vi "getcalpwr.vi"(5 "RF On":bool=TRUE, 7 "caldata":dbl[][](array[numeric]) format="%0.3f", 8 "RF HP":bool=TRUE, 9 "attn":dbl, 10 "freq":dbl=1000.0 min=34.375 max=4400.0 step=1.0 format="%_7g") -> (2 "actual":dbl)   [LabVIEW 2012]
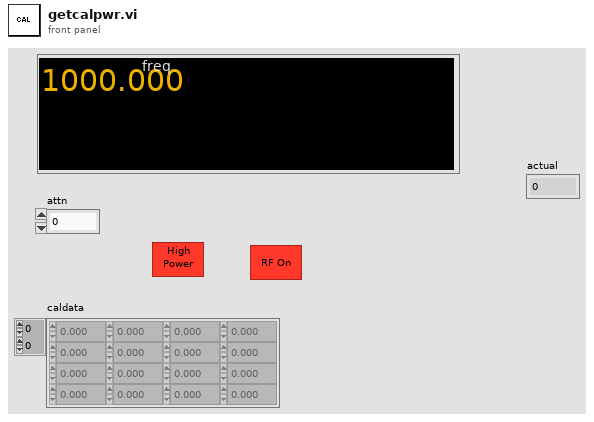
[diagram p1: front panel]
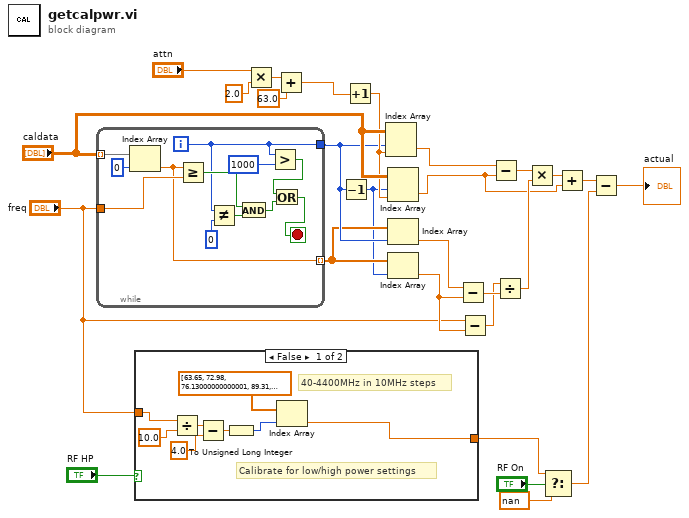
[diagram p0: block diagram]
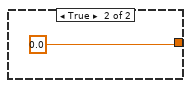
[diagram p2: hidden frame]
diagram:
  n1 = while {
    tunnel: "caldata" -> [w39] mode=indexing
    tunnel: "freq" -> [w37]
    tunnel: [w32] -> w25
    tunnel: [w33] -> w24 mode=indexing
    i -> [w32]
    stop <- w28 stop-if-true
    n2 = Index Array(array=w39, index=0) -> (element=w33:dbl)
    n3 = Greater Or Equal?(x=w33, y=w37) -> (x >= y?=w34:bool)
    n4 = Not Equal?(x=w32, y=0) -> (x != y?=w35:bool)
    n5 = And(x=w34, y=w35) -> (x .and. y?=w30:bool)
    n6 = Greater?(x=w32, y=1000) -> (0:w29:bool)
    n7 = Or(x=w29, y=w30) -> (x .or. y?=w28:bool)
  }
  n8 = case shown="False" "RF HP" {
    tunnel: [w40 0.0] -> w8
    tunnel: "freq" -> [w46 _]
    frame False {
      # "Calibrate for low/high power settings"
      # "40-4400MHz in 10MHz steps"
      n9 = Divide(x=w46, y=10.0) -> (x/y=w44:dbl)
      n10 = Subtract(x=w44, y=4.0) -> (x-y=w42:dbl)
      n11 = To Unsigned Long Integer(number=w42) -> (unsigned 32bit integer=w41:u32)
      n12 = Index Array(array=dbl[] [63.65, 72.98, 76.13000000000001, 89.31, 77.55000000000001, 78.89, 84.86, 81.81, 79.77000000000001, 80.12, 77.53, 78.39000000000001, 76.36, 76.32, 75.96, 74.75999999999999, 74.81, 74.34, 73.81, 73.35, 72.8, 72.87, 72.71000000000001, 71.77, 71.39, 71.28, 71.19, 70.59, 70.28, 69.9, 70.14999999999999, 69.73, 69.03, 69.1, 69.16, 68.39, 68.81, 67.9, 67.76, 67.55, 67.13, 67.02, 66.84, 66.67, 66.37, 66.11, 65.95, 65.74000000000001, 65.41, 65.23, 65.15, 64.83, 64.59, 64.46, 64.36, 64.14, 63.99, 63.79, 63.64, 63.53, 63.39, 63.18000000000001, 63.02, 62.88, 62.8, 62.63, 62.489999999999995, 62.349999999999994, 62.17999999999999, 62.019999999999996, 61.86, 61.699999999999996, 61.620000000000005, 61.53, 61.46, 61.3, 61.2, 61.120000000000005, 60.910000000000004, 60.730000000000004, 60.68, 60.56, 60.510000000000005, 60.440000000000005, 60.26, 59.98, 59.98, 59.8, 59.75, 59.589999999999996, 59.559999999999995, 59.43, 59.29, 59.290000000000006, 59.1, 59.019999999999996, 58.95, 58.92, 58.82, 58.82, 58.68, 58.52, 58.519999999999996, 58.56, 58.44, 58.32, 58.44, 58.349999999999994, 58.3, 58.25, 58.089999999999996, 58.0, 57.97, 57.97, 57.89, 57.86, 57.81999999999999, 57.769999999999996, 57.65, 57.510000000000005, 57.480000000000004, 57.38, 57.27, 57.26, 57.120000000000005, 57.089999999999996, 57.07, 57.07, 56.93, 56.85, 56.9, 56.84, 56.72, 56.74, 56.56, 56.44, 56.45, 56.35, 56.35, 56.3, 56.300000000000004, 56.330000000000005, 56.18, 55.989999999999995, 56.0, 55.83, 55.870000000000005, 56.0, 55.81, 55.53, 55.690000000000005, 55.85, 55.599999999999994, 55.36, 55.57, 55.86, 55.63, 55.24, 55.48, 55.72, 55.22, 55.56, 55.18000000000001, 54.790000000000006, 55.11, 54.79, 55.05, 54.72, 54.83, 54.93, 54.709999999999994, 54.48, 54.64, 54.53, 54.64, 54.53, 54.53, 54.42, 54.39, 54.339999999999996, 54.27, 54.34, 54.39, 54.25, 54.3, 54.22, 54.06, 54.089999999999996, 54.21, 54.31, 54.24, 54.14, 54.14, 54.11, 53.8, 53.830000000000005, 53.68, 53.53, 53.6, 53.519999999999996, 53.66, 53.47, 53.5, 53.410000000000004, 53.489999999999995, 53.510000000000005, 53.580000000000005, 53.550000000000004, 53.540000000000006, 53.49, 53.49, 53.34, 53.2, 53.17, 53.14, 53.080000000000005, 47.42, 47.03, 46.699999999999996, 46.56, 46.449999999999996, 46.31, 45.980000000000004, 45.89, 45.790000000000006, 45.739999999999995, 45.43, 45.120000000000005, 45.01, 44.89, 44.71, 44.33, 44.29, 44.120000000000005, 44.04, 43.72, 43.51, 43.480000000000004, 43.46, 43.39, 43.09, 42.96, 42.93, 42.93, 42.74, 42.44, 42.41, 42.48, 42.54, 42.4, 42.150000000000006, 42.17, 42.290000000000006, 42.31, 42.15, 41.96, 41.93, 41.89, 41.87, 41.71, 41.47, 41.48, 41.47, 41.45, 41.230000000000004, 40.89, 40.81, 40.67, 40.58, 40.5, 40.230000000000004, 40.04, 40.0, 39.79, 39.68, 39.49, 39.22, 39.11, 39.059999999999995, 38.85, 38.7, 38.44, 38.28, 38.15, 43.05, 43.150000000000006, 43.11, 43.08, 42.75, 42.57, 42.72, 42.88, 42.94, 42.72, 42.83, 42.89, 43.04, 43.089999999999996, 42.83, 42.86, 42.93, 43.0, 42.99, 42.940000000000005, 42.519999999999996, 42.39, 42.37, 42.28, 42.41, 41.86, 42.06, 42.129999999999995, 42.3, 42.44, 42.540000000000006, 41.9, 41.95, 41.91, 42.05, 42.16, 42.129999999999995, 41.370000000000005, 41.37, 41.4, 41.540000000000006, 41.82, 41.919999999999995, 41.88, 41.15, 41.17, 41.3, 41.489999999999995, 41.669999999999995, 41.68, 40.85, 40.83, 40.78, 40.76, 40.8, 40.82, 40.73, 39.81, 39.76, 39.72, 39.76, 39.95, 40.07, 40.099999999999994, 39.37, 39.410000000000004, 39.43, 39.42, 39.5, 39.54, 39.519999999999996, 39.379999999999995, 38.53, 38.400000000000006, 38.35, 38.31, 38.38, 38.35, 38.260000000000005, 38.169999999999995, 46.31, 46.379999999999995, 46.48, 46.6, 46.83, 47.55, 47.98, 48.57, 49.36, 50.62, 53.26, 56.38999999999999, 62.22, 69.38, 57.89, 50.67, 47.5, 45.5, 43.83, 42.53, 41.1, 40.32, 39.669999999999995, 39.04, 38.449999999999996, 37.84, 37.03, 36.58, 36.18, 35.849999999999994, 35.57, 35.31, 34.75, 34.63, 34.59, 34.57, 34.69, 34.62, 34.919999999999995, 35.099999999999994, 35.49, 35.739999999999995, 36.18, 36.3, 36.870000000000005, 37.38, 37.89, 38.48, 39.18, 39.9, 40.18, 40.83, 41.43, 42.03, 42.64, 43.12, 43.39, 43.83, 44.309999999999995, 44.67, 44.94, 45.0, 44.96, 44.809999999999995, 44.709999999999994, 44.660000000000004, 44.64, 44.48, 44.190000000000005, 44.02, 43.830000000000005, 43.78, 43.67] ("Delta"), index=w41) -> (element=w40:dbl)
    }
    frame True {
    }
  }
  n13 = Multiply(x="attn", y=2.0) -> (x*y=w5:dbl)
  n14 = Add(x=w5, y=63.0) -> (x+y=w2:dbl)
  n15 = Decrement(x=w25) -> (x-1=w23:i32)
  n16 = Increment(x=w2) -> (x+1=w26:dbl)
  n17 = Index Array(array="caldata", index (row)=w25, index (col)=w26) -> (element=w18:dbl)
  n18 = Index Array(array="caldata", index (row)=w23, index (col)=w26) -> (element=w14:dbl)
  n19 = Index Array(array=w24, index=w25) -> (element=w22:dbl)
  n20 = Index Array(array=w24, index=w23) -> (element=w21:dbl)
  n21 = Subtract(x=w22, y=w21) -> (x-y=w20:dbl)
  n22 = Subtract(x="freq", y=w21) -> (x-y=w19:dbl)
  n23 = Subtract(x=w18, y=w14) -> (x-y=w17:dbl)
  n24 = Divide(x=w19, y=w20) -> (x/y=w16:dbl)
  n25 = Multiply(x=w17, y=w16) -> (x*y=w15:dbl)
  n26 = Select(t=w8, s="RF On", f=nan) -> (s? t:f=w7:dbl)
  n27 = Add(x=w15, y=w14) -> (x+y=w13:dbl)
  n28 = Subtract(x=w13, y=w7) -> (x-y=→"actual":dbl)
